vi "Pixy_COM-RIO.vi"() -> ()   [LabVIEW 2016]
uses:
  <vilib>/Analysis/baseanly.llb/Mean (DBL).vi
  <vilib>/Instr/_visa.llb/VISA Configure Serial Port (Instr).vi
  <vilib>/Analysis/NI_AALBase.lvlib
panel:
  out "Data out":T1
  out "Initialization error out":errorcluster
  out "Read error out":errorcluster
  out "X":i32
  out "Y":i32
  out "Width":i32
  out "Height":i32
  out "Area":dbl(graph)
  in  "Command":string(combo)
  in  "Write Command?":bool
  in  "Display buffer size":u16=100 min=1
  out "Data display":string
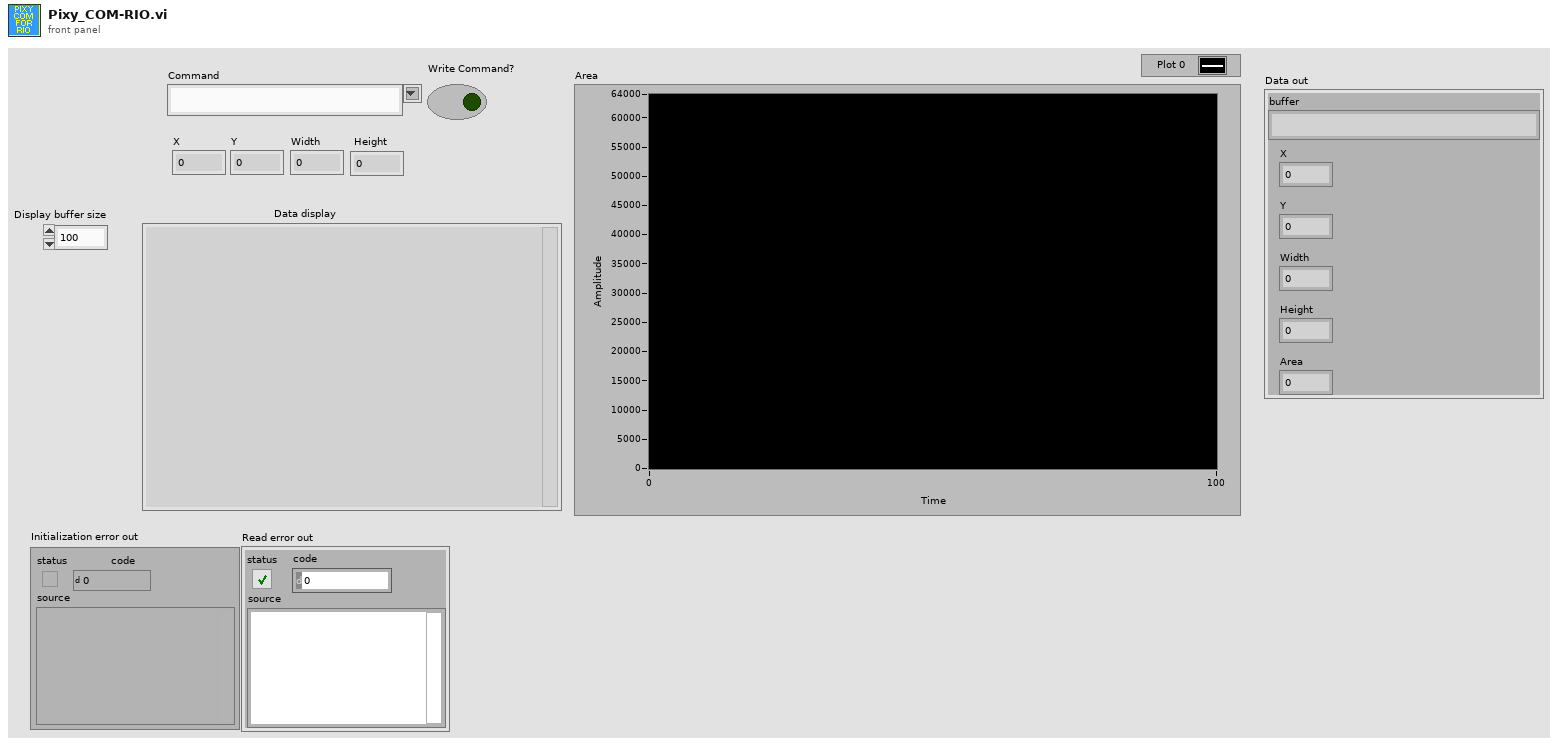
[diagram p1: front panel]
types:
  T1 = cluster{"buffer":string, "X":i32, "Y":i32, "Width":i32, "Height":i32, "Area":dbl}
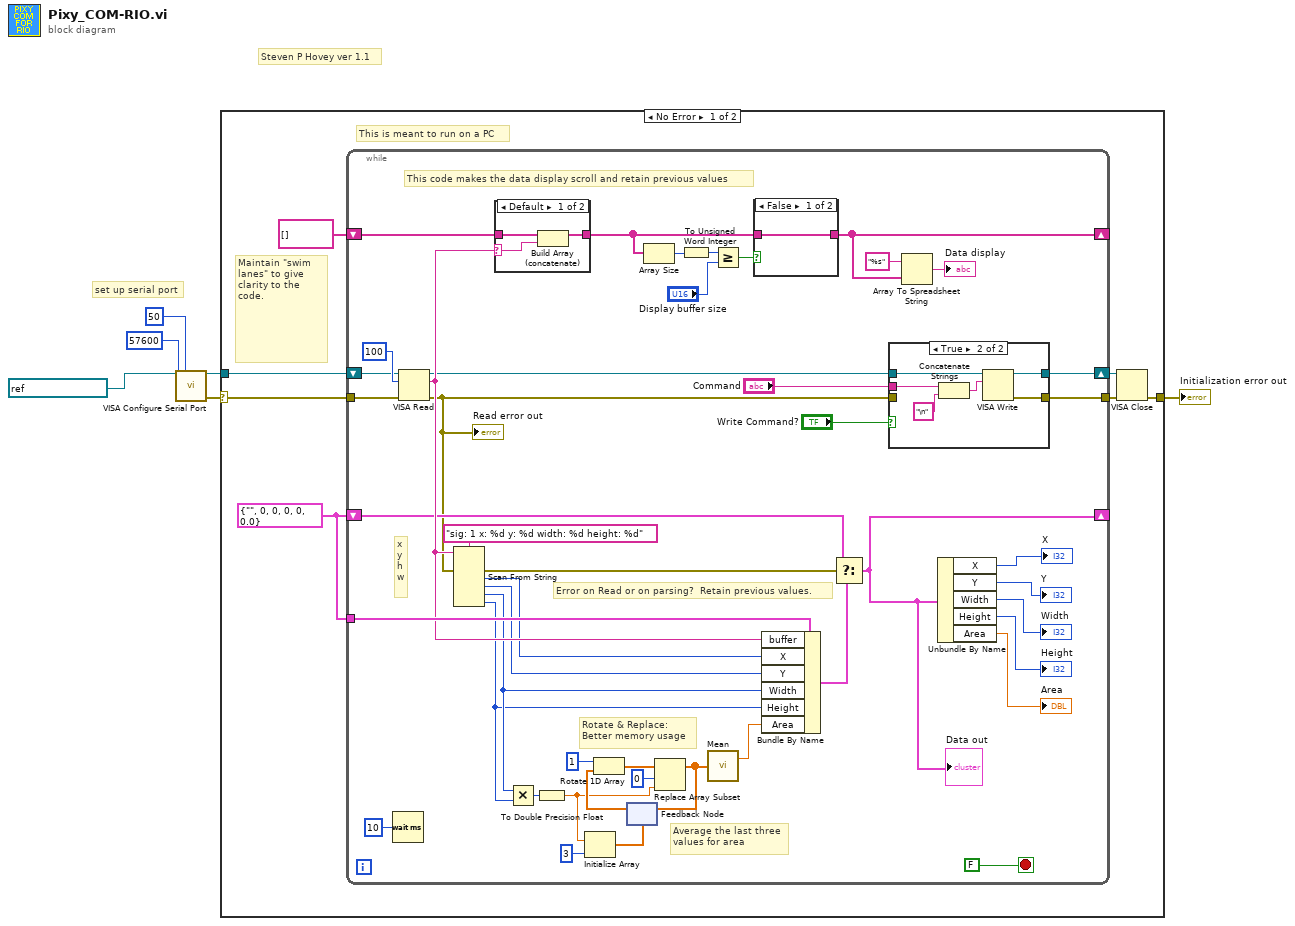
[diagram p0: block diagram]
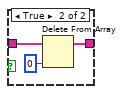
[diagram p3: hidden frame]
diagram:
  # "Steven P Hovey ver 1.1"
  # "set up serial port"
  n1 = call-poly "VISA Configure Serial Port"("VISA resource name"=refnum<visa-resource-name> "ASRL4::INSTR", "timeout (10sec)"=u32 50, "baud rate (9600)"=u32 57600) -> ("VISA resource name out"=w4:refnum<visa-resource-name>, "error out"=w2:errorcluster)  [unwired: 11 in]
  n2 = case shown="No Error" w2 {
    selector: w2 -> [w7 w76]
    tunnel: w4 -> [w13 _]
    tunnel: [w8 w76] -> w3
    frame No Error {
      w11 = T1 {"buffer"="", "X"=0, "Y"=0, "Width"=0, "Height"=0, "Area"=0.0}
      # "Maintain \"swim lanes\" to give clarity to the code."
      # "This is meant to run on a PC"
      n3 = while {
        shift-right: [w48] -> w10
        shift-left: w13 -> [w55]
        shift-right: [w30] -> _
        shift-left: w11 -> [w32]
        shift-right: [w24] -> _
        shift-left: string[] [] -> [w45]
        tunnel: w11 -> [w59]
        tunnel: w7 -> [w21]
        tunnel: [w22] -> w9
        stop <- FALSE ("stop") stop-if-true
        # "Error on Read or on parsing?  Retain previous values."
        # "Rotate & Replace:\nBetter memory usage"
        # "Average the last three\nvalues for area"
        # "This code makes the data display scroll and retain previous values"
        # "x\ny\nh\nw"
        n4 = Wait (ms)(milliseconds to wait=u32 10) -> ()  [unwired: 1 out]
        n5 = VISA Read(VISA resource name=w55, byte count=u32 100, error in (no error)=w21) -> (VISA resource name out=w49:refnum<visa-resource-name>, read buffer=w58:string, error out=w19:errorcluster)  [unwired: 1 out]
        "Read error out" <- w19
        n6 = Scan From String(format string="sig: 1 x: %d y: %d width: %d height: %d", input string=w58, error in=w19) -> (error out=w33:errorcluster, output 1=w38:i32, output 2=w37:i32, output 3=w36:i32, output 4=w35:i32)  [unwired: 5 in, 2 out]
        n7 = case shown="Default" w58 {
          selector: w58 -> [w60 _]
          tunnel: w45 -> [w61 w63]
          tunnel: [w62 w63] -> w25
          frame Default {
            n8 = Build Array (concatenate)(w61, w60) -> (w62:string[])
          }
          frame "" {
          }
        }
        n9 = Multiply(x=w36, y=w35) -> (x*y=w34:i32)
        n10 = To Double Precision Float(number=w34) -> (double precision float=w26:dbl)
        n11 = Initialize Array(w26, 3 ("dimension size")) -> (w52:dbl[])
        n12 = feedback #1(w52) -> (w29:dbl[])
        n13 = Rotate 1D Array(1:w29, 2:1 ("n")) -> (0:w28:dbl[])
        n14 = Array Size(array=w25) -> (size(s)=w43:i32)
        n15 = Replace Array Subset(array=w28, new element=w26, index=0) -> (w51:dbl[])
        n16 = feedback-in #1(w51) -> ()
        n17 = To Unsigned Word Integer(number=w43) -> (unsigned 16bit integer=w42:u16)
        n18 = call-poly <vilib>:"Mean.vi"("X"=w51) -> ("mean"=w54:dbl)  [unwired: 1 out]
        n19 = Greater Or Equal?(x=w42, y="Display buffer size") -> (x >= y?=w41:bool)
        n20 = case shown="False" w41 {
          tunnel: w25 -> [w64 w67]
          tunnel: [w64 w66] -> w24
          frame False {
          }
          frame True {
            n21 = Delete From Array(array=w67, index=0) -> (array with subset deleted=w66:string[])  [unwired: 1 in, 1 out]
          }
        }
        n22 = Bundle By Name(cluster=w59, "buffer"=w58, "X"=w38, "Y"=w37, "Width"=w36, "Height"=w35, "Area"=w54) -> (w31:T1)
        n23 = Select(t=w32, s=w33, f=w31) -> (s? t:f=w30:T1)
        "Data out" <- w30
        n24 = case shown="True" "Write Command?" {
          tunnel: w49 -> [w69 w75]
          tunnel: [w69 w74] -> w48
          tunnel: "Command" -> [_ w73]
          tunnel: w19 -> [w68 _]
          tunnel: [w68 w72] -> w22
          frame False {
          }
          frame True {
            n25 = Concatenate Strings(w73, "\n") -> (w71:string)
            n26 = VISA Write(VISA resource name=w75, write buffer=w71) -> (VISA resource name out=w74:refnum<visa-resource-name>, error out=w72:errorcluster)  [unwired: 1 in, 1 out]
          }
        }
        n27 = Array To Spreadsheet String(array=w24, 3:"%s" ("format string")) -> (spreadsheet string=→"Data display":string)  [unwired: 1 in]
        n28 = Unbundle By Name(w30) -> ("X"=→"X":i32, "Y"=→"Y":i32, "Width"=→"Width":i32, "Height"=→"Height":i32, "Area"=→"Area":dbl)
      }
      n29 = VISA Close(VISA resource name=w10, error in (no error)=w9) -> (error out=w8:errorcluster)
    }
    frame Error {
    }
  }
  "Initialization error out" <- w3
